vi "Read Field Polynomial.vi"(8 "error in (no error)":errorcluster, 11 "input cluster":T1) -> (0 "error out":errorcluster, 2 "Field (T)":dbl, 3 "output cluster":T1)   [LabVIEW 2012]
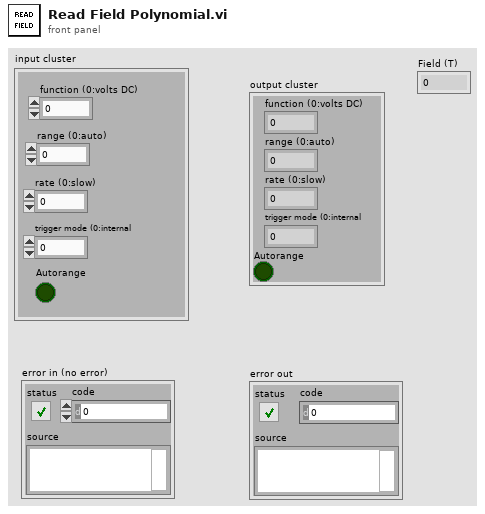
[diagram p1: front panel]
types:
  T1 = cluster{"function (0:volts DC)":i16, "range (0:auto)":i16, "rate (0:slow)":i16, "trigger mode (0:internal":i16, "Autorange":bool}
  T2 = cluster{"function (0:volts DC)":u16, "range (0:auto)":u16, "rate (0:slow)":u16, "trigger mode (0:internal)":u16, "Autorange":bool}
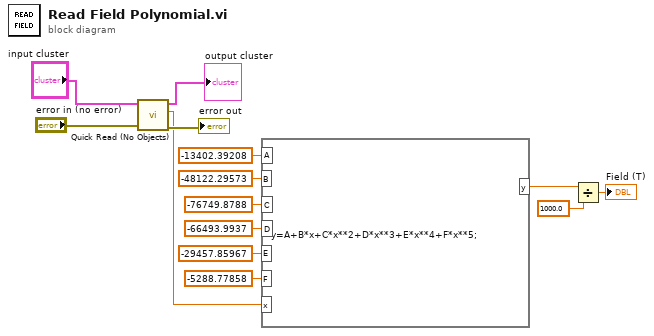
[diagram p0: block diagram]
diagram:
  n1 = call "Quick Read (No Objects).vi"("error in (no error)"="error in (no error)", "Fluke Multimeter In"="input cluster") -> ("error out"=→"error out":errorcluster, "measurement"=w4:dbl, "Fluke Multimeter Out"=→"output cluster":T2)  [unwired: 6 in, 1 out]
  n2 = formula code="y=A+B*x+C*x**2+D*x**3+E*x**4+F*x**5;"("A"=-13402.39208 ("input variable"), "B"=-48122.29573 ("input variable"), "C"=-76749.8788 ("input variable"), "D"=-66493.9937 ("input variable"), "E"=-29457.85967 ("input variable"), "F"=-5288.77858 ("input variable"), "x"=w4) -> ("y"=w2:dbl)
  n3 = Divide(x=w2, y=1000.0 ("x")) -> (x/y=→"Field (T)":dbl)
